vi "Write Resampler Configuration.vi"(8 "error in (no error)":errorcluster, 10 "Resampler Configuration":T1={"Group"="p", "Reference channel"="", "Channels to resample"=[]}, 11 "Resampler in":refnum<class "Resampler.lvclass">) -> (0 "error out":errorcluster, 3 "Resampler out":refnum<class "Resampler.lvclass">)   [LabVIEW 2024, in "Resampler.lvclass"]
uses:
  Resampler.lvclass
  C:/Nano/fedor2024/labview/LabActor/Template Module/Template Module.lvclass
  Resampler Configuration.ctl
  Template Module/Template Module.lvclass/Template Module.ctl
  Template Module/Write Configuration.vi
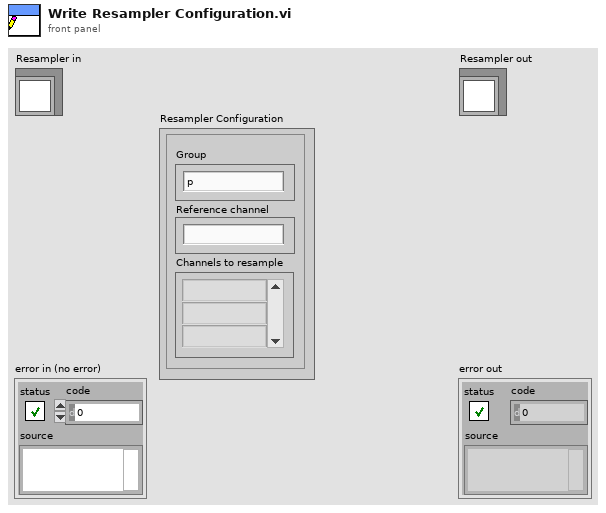
[diagram p1: front panel]
types:
  T1 = typedef "Resampler Configuration.ctl" = cluster{"Group":string, "Reference channel":string, "Channels to resample":string[]}
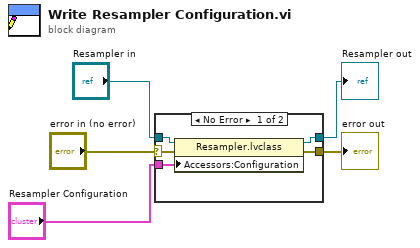
[diagram p0: block diagram]
diagram:
  n1 = case shown="No Error" "error in (no error)" {
    selector: "error in (no error)" -> [w8 w11]
    tunnel: [w9 w11] -> w4
    tunnel: [w6 w12] -> w2
    tunnel: "Resampler in" -> [w7 w12]
    tunnel: "Resampler Configuration" -> [w10 _]
    frame No Error {
      n2 = property class="Resampler.lvclass"(reference=w7, error in=w8, "Accessors:Configuration"=w10) -> (reference out=w6:refnum<class "Resampler.lvclass">, error out=w9:errorcluster)
    }
    frame Error {
    }
  }
  "error out" <- w4
  "Resampler out" <- w2
